vi "Test Skip Overrides Downstreams Error Status.vi"(8 "error in (no error)":errorcluster, 11 "Test Assertion Results in":refnum<class "Assertion Result Test.lvclass">) -> (0 "error out":errorcluster, 3 "Test Assertion Results out":refnum<class "Assertion Result Test.lvclass">)   [LabVIEW 2020, in "LUnit Tests.lvlib" / "Assertion Result Test.lvclass"]
uses:
  Assertion Result Test.lvclass
  C:/Program Files (x86)/National Instruments/LabVIEW 2020/vi.lib/Astemes/LUnit/Test Case.lvclass
  Test Dummys/Test Case Test Double/Test Case Test Double.lvclass
  C:/Git/astemes-lunit/source/Framework/Test Case/LUnit Test Case.lvclass
  source/Framework/Result Types/Assertion Result/Public/TypeDefs/Status.ctl
  source/Framework/Test Case/LUnit Test Case.lvclass/LUnit Test Case.ctl
  <vilib>/Astemes/LUnit/Test Case.lvclass/Test Case.ctl
  source/Framework/Result Types/Case Result/Private/Merge Status.vi
  <vilib>/Astemes/LUnit/Palette/Fail.vi
  <vilib>/Astemes/LUnit/Palette/Pass.vi
  <vilib>/Astemes/LUnit/Set Assertion Type.vi
  <vilib>/Astemes/LUnit/Add test result.vi
  <vilib>/Astemes/LUnit/LUnit Record Assertion Result.vi
  <vilib>/Astemes/LUnit/LUnit Aggregate Assertion Results.vi
  <vilib>/Astemes/LUnit/Method Result/LUnit Merge Status.vi
  <vilib>/Astemes/LUnit/LUnit Concatenate result strings.vi
  source/Framework/Test Case/LUnit Test Case.lvclass
  source/Framework/Result Types/Case Result/Test Case Result.lvlib
  <vilib>/Astemes/LUnit/Test Case.lvclass
  source/Framework/Result Types/Assertion Result/Assertion Result.lvlib
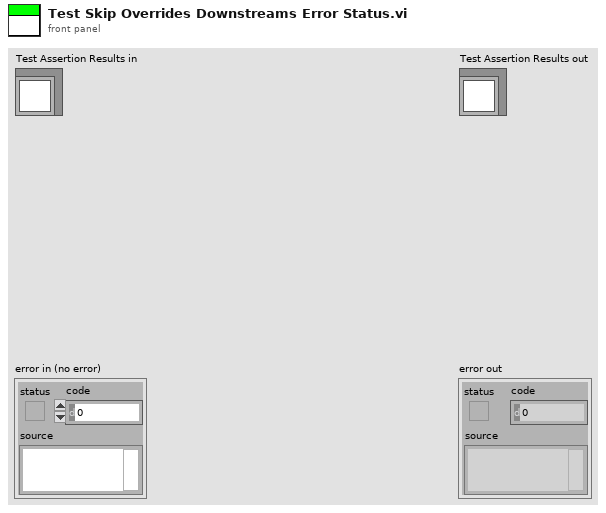
[diagram p1: front panel]
types:
  T1 = typedef "Assertion Result.lvlib/Status.ctl" = enum16{"Pass", "Fail", "Error", "Skipped", "Setup Error", "Broken", "Teardown Error"}
  T2 = typedef "Test Case Result.lvlib/Test Case Result type.ctl" = map{string, T3}
  T3 = typedef "Method Result.lvlib/Method Result type.ctl" = cluster{"Test Case":string, "Test Method Name":string, "Status":T1, "Assertion Results":T4[], "Execution time":dbl, "Result String":string}
  T4 = typedef "Assertion Result.lvlib/Assertion Result type.ctl" = cluster{"Status":T1, "Message":string, "Description":string, "Assertion Type":T5}
  T5 = typedef "Assertion Result.lvlib/Assertion Type.ctl" = enum16{"None", "Pass", "Fail", "Skip", "Pass if Equal", "Fail if Equal", "Pass if Error", "Fail if Error", "Pass if", "Fail if"}
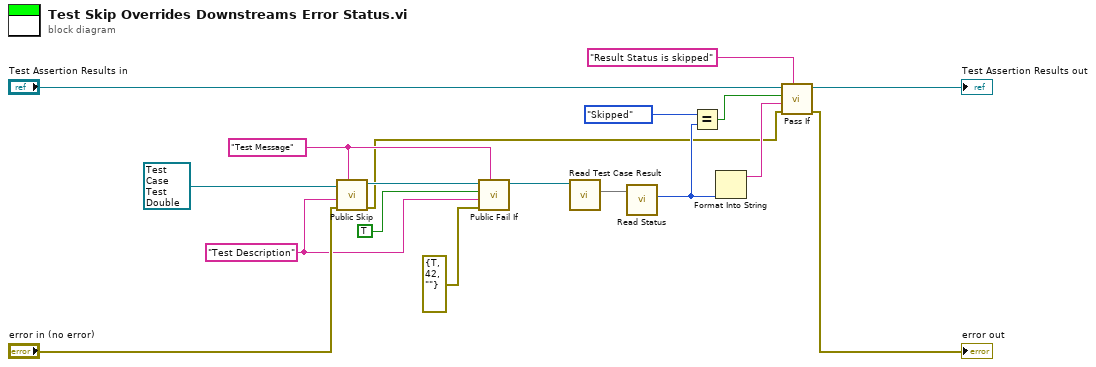
[diagram p0: block diagram]
diagram:
  w3 = "Test Message" ("Description")
  w4 = "Test Description" ("Description")
  n1 = call "Public Skip.vi"("Description"=w3, "error in (no error)"="error in (no error)", "Message"=w4, "Test Case Test Double in"=refnum<class "Test Case Test Double.lvclass"> refnum ("Test Case Test Double.lvclass")) -> ("error out"=w1:errorcluster, "Test Case Test Double out"=w7:refnum<class "Test Case Test Double.lvclass">)  [unwired: 6 in]
  n2 = call "Public Fail If.vi"("Message"=w3, "error in (no error)"=errorcluster {"status"=TRUE, "code"=42, "source"=""}, "Description"=w4, "Fail?"=TRUE, "Test Case Test Double in"=w7) -> ("Test Case Test Double out"=w6:refnum<class "Test Case Test Double.lvclass">)  [unwired: 5 in, 1 out]
  n3 = call "Read Test Case Result.vi"("LUnit Test Case In"=w6) -> ("Test Case Result"=w15:T2)  [unwired: 9 in, 1 out]
  n4 = call "Read Status.vi"("Test Case Result In"=w15) -> ("Status"=w10:T1)  [unwired: 8 in, 2 out]
  n5 = Equal?(x=Status."Skipped" ("y"), y=w10) -> (x = y?=w8:bool)
  n6 = Format Into String(w10) -> (resulting string=w12:string)  [unwired: 3 in, 1 out]
  n7 = call <vilib>:"Pass If.vi"("Description"="Result Status is skipped", "error in (no error)"=w1, "Message"=w12, "Pass?"=w8, "LUnit Test Case In"="Test Assertion Results in") -> ("error out"=→"error out":errorcluster, "LUnit Test Case Out"=→"Test Assertion Results out":refnum<class "Assertion Result Test.lvclass">)  [unwired: 5 in]
